vi "AlliGator Init Image Profile Window Menu.vi"(8 "error in":errorcluster, 11 "Menu in":refnum<k9>) -> (0 "error out":errorcluster)   [LabVIEW 2021, in "AlliGator Image Profile Window.lvlib"]
doc: "Initialize Profile Window menu."
uses:
  AlliGator Image Profile Window.lvlib
  AlliGator Variables List.ctl
  Image/Box Profile Type.ctl
  AlliGator Image Profile Intensity Type.ctl
  AlliGator Image Profile Average Intensity Type.ctl
  Variant/Variant to Data/Variant to Boolean.vi
  AlliGator Globals, Variables & Constants.lvlib
  Variant/Variant to Data/Variant to Data.lvlib
  Image/Image.lvlib
panel:
  # "see the AlliGator License on the block diagram (Ctrl+E or Window:Show Block Diagram)"
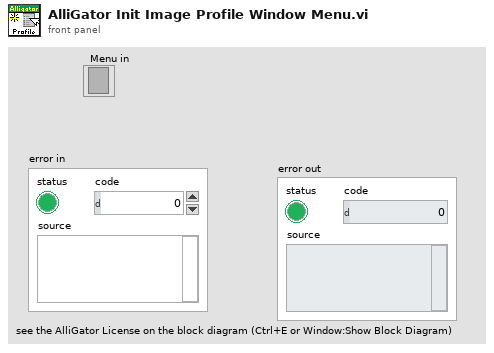
[diagram p1: front panel]
types:
  T1 = typedef "AlliGator Image Profile Window.lvlib/AlliGator Image Profile Average Intensity Type.ctl" = enum16{"Integrated Intensity", "Average Intensity", "Intensity-weighted Average Intensity"}
  T2 = typedef "AlliGator Image Profile Window.lvlib/AlliGator Image Profile Intensity Type.ctl" = enum16{"Raw Data", "Displayed Image", "Background-subtracted"}
  T3 = typedef "AlliGator Globals, Variables & Constants.lvlib/AlliGator Variables List.ctl" = enum16{"---- GUI ----", "Initialization Status", "State Indicators Refnum", "Original AlliGator Menu Items", "Current Action Loop State", "Script in progress", "Playback", "Loop Playback", "Search ROI Used", "Search ROI", "Decay Graph Max Legend Size", "Intensity Graph Max Legend Size", "Decay Statistics Graph Max Legend Size", "Phasor Graph Max Legend Size", "Phasor Ratio Graph Max Legend Size", "Lifetime Graph Max Legend Size", "---- Files ----", "Export Dataset Frames as Individual Files", "Show Batch Export Help Balloons", "Frames in Dataset", "ptu File Frame Start Indices", "Current Frame in Dataset", "Current Frame Timestamp", "------ Python Plugins ------", "Python Plugins Information", "Python Session", "Valid Python Session?", "---- Source Image ----", "Dataset Loaded", "Dataset Metadata", "Dataset Channel", "Dataset Data Description", "Background Dataset Metadata", "Background Dataset Channel", "Background Dataset Data Description", "Background File Subtraction", "Background File Path", "Background File Pile-up Correction", "Background File Pixel Well Capacity", "Background File Scaling Factor", "Source Image ROIs", "Current Source Image ROI", "Source Image ROI Event Refnum", "X_Source Image Display Range", "X_Source Image Palette Information", "Source Image Palette List", "Source Image Scale", "Current Dataset Load Settings", "Source Image:ROI Overlay Color", "---- Image Profile Window ----", "Image Profile:Overlay ROI in Source Image", "Image Profile Window Event Refnum", "Image Profile:IntensityType", "Image Profile:Intensity Average Type", "Image Profile:Intensity-weighted SDV", "Image Profile:Box Profile Type", "Image Profile Window Open", "Image Profile:Plotted Fit Parameter", "X_Type of Displayed Image", "X_Time Gate Slider", "Dataset Path", "Source Image Overlay to Erase", "Is Displayed Image Accumulated", "White Light Image Modified", "Mask Image Modified", "Macrotime Gate Separation", "------ Phasor Graph -------", "Phasor Graph:Show Line", "---- Phasor Plot ---", "Phasor Plot Parameters Changed", "FLI Dataset Modified since last Phasor Plot Calculation", "Phasor Harmonics Data", "Selected Phasor Harmonics", "Phasor Harmonic Manager Event Refnum", "Phasor Plot ROIs", "Current Phasor Plot ROI", "Phasor Plot ROI Event Refnum", "Phasor Plot Image Reference Points", "Phasor Plot Computed", "Phasor Plot Palette Information", "Phasor Plot Palette List", "Phasor Ratio Palette Information", "Phasor Ratio Palette List", "Phasor Image Scale", "Phasor Plot Image Overlay to Erase", "Phasor Plot Image Elements to Update", "Current Phasor Plot Calculation Parameters", "Current Phasor Calibration Options", "Reset Cumulated Phasor Plot", "Phasor Ratio Reference 1", "Phasor Ratio Lifetime Reference 1", "Phasor Ratio Reference 1 Frequency", "Phasor Ratio Reference 2", "Phasor Ratio Lifetime Reference 2", "Phasor Ratio Reference 2 Frequency", "---- Decay Analysis ----", "Number of Selected Decays to Fit", "LS Fit Results", "LAR Fit Results", "BS Fit Results", "Last Decay Max - Min", "Best Fit Parameters", "Best Fit Parameter Names", "Actual Size X", "Actual Size Y", "Binning X", "Binning Y", "Actual # Gates", "Dataset Number", "Gates to...", "Gates Skipped", "Gates to keep", "Gate Step", "Gate Separation", "Reversed Gates", "Pile-up Correction", "Pixel Well Capacity", "Background Subtracted", "Background Subtraction Method", "Background Definition Range", "Background File (deprecated)", "Number of Dataset Accumulated", "Array of Accumulated Dataset Paths", "Do Averaged Datasets", "Destination File Path", "Process Plot Target", "Use 1/D as Phasor Frequency", "---- Decay Fit Parameter Map -----", "Decay Fit Parameter Map Palette Information", "Decay Fit Parameter Map Palette List", "Local Decay Graph Window Event Refnum", "------- Local Decay Window ---------", "Use normalized IRF for convolution", "----- Miscellaneous ----", "Skippable Dialog Windows Status"}
  T4 = typedef "Image.lvlib/Box Profile Type.ctl" = enum16{"Full Width", "Half Width"}
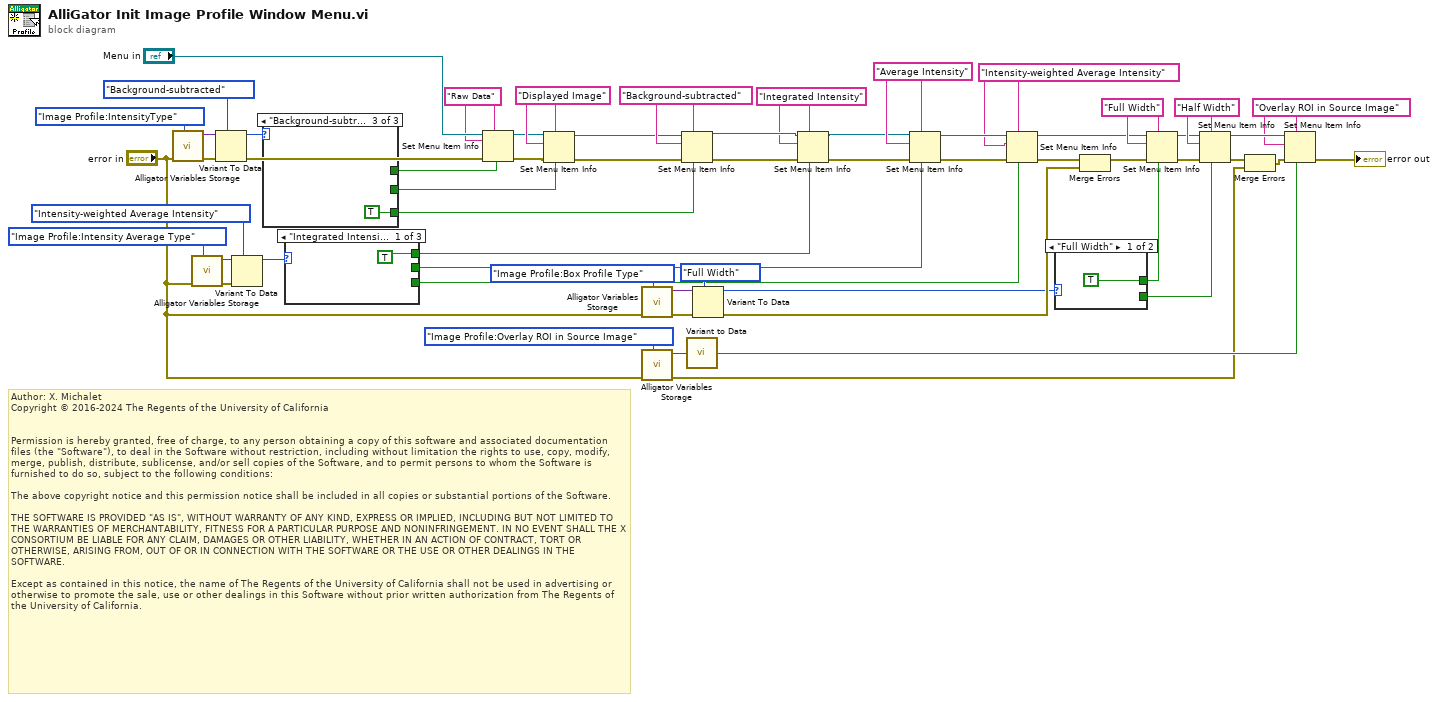
[diagram p0: block diagram]
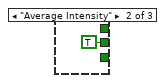
[diagram p2: hidden frame]
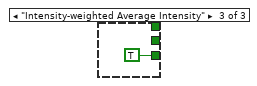
[diagram p3: hidden frame]
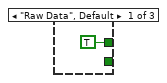
[diagram p4: hidden frame]
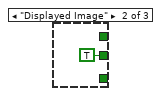
[diagram p5: hidden frame]
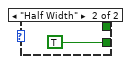
[diagram p6: hidden frame]
diagram:
  w2 = "Integrated Intensity" ("item tag")
  w13 = "Intensity-weighted Average Intensity" ("ItemTag")
  w14 = "Average Intensity" ("ItemTag")
  w34 = "Overlay ROI in Source Image" ("item tag")
  w55 = "Half Width" ("item tag")
  w54 = "Full Width" ("item tag")
  w50 = "Background-subtracted" ("ItemTag")
  w40 = "Raw Data" ("ItemTag")
  w41 = "Displayed Image" ("ItemTag")
  # "Author: X. Michalet\nCopyright © 2016-2024 The Regents of the University of California\n \n\nPermission is hereby granted, free of charge, to any person obtaining a copy of this software and associated documentation files (the \"Software\"), to deal in the Software without restriction, including without limitation the rights to use, copy, modify, merge, publish, distribute, sublicense, and/or sell copies of the Software, and to permit persons to whom the Software is furnished to do so, subject to the following conditions:\n\nThe above copyright notice and this permission notice shall be included in all copies or substantial portions of the Software.\n\nTHE SOFTWARE IS PROVIDED \"AS IS\", WITHOUT WARRANTY OF ANY KIND, EXPRESS OR IMPLIED, INCLUDING BUT NOT LIMITED TO THE WARRANTIES OF MERCHANTABILITY, FITNESS FOR A PARTICULAR PURPOSE AND NONINFRINGEMENT. IN NO EVENT SHALL THE X CONSORTIUM BE LIABLE FOR ANY CLAIM, DAMAGES OR OTHER LIABILITY, WHETHER IN AN ACTION OF CONTRACT, TORT OR OTHERWISE, ARISING FROM, OUT OF OR IN CONNECTION WITH THE SOFTWARE OR THE USE OR OTHER DEALINGS IN THE SOFTWARE.\n\nExcept as contained in this notice, the name of The Regents of the University of California shall not be used in advertising or otherwise to promote the sale, use or other dealings in this Software without prior written authorization from The Regents of the University of California."
  n1 = call "Alligator Variables Storage.vi"("AlliGator Variable"=AlliGator_Variables_List."Image Profile:IntensityType" ("Alligator Variable"), "Error In"="error in") -> ("Error Out"=w38:errorcluster, "Data out"=w24:variant)  [unwired: 7 in, 1 out]
  n2 = call "Alligator Variables Storage.vi"("AlliGator Variable"=AlliGator_Variables_List."Image Profile:Intensity Average Type" ("Alligator Variable"), "Error In"="error in") -> ("Error Out"=w11:errorcluster, "Data out"=w12:variant)  [unwired: 7 in, 1 out]
  n3 = Variant To Data(error in=w38, type=AlliGator_Image_Profile_Intensity_Type."Background-subtracted" ("Image Profile Intensity Type"), Variant=w24) -> (data=w22:T2, error out=w25:errorcluster)
  n4 = Variant To Data(error in=w11, type=AlliGator_Image_Profile_Average_Intensity_Type."Intensity-weighted Average Intensity" ("Image Profile Average Intenisty Type"), Variant=w12) -> (data=w10:T1)  [unwired: 1 out]
  n5 = case shown="\"Background-subtracted\"" w22 {
    tunnel: [TRUE ("checked") _ _] -> w21
    tunnel: [_ TRUE ("checked") _] -> w20
    tunnel: [_ _ TRUE ("checked")] -> w19
    frame "Raw Data", Default {
    }
    frame "Displayed Image" {
    }
    frame "Background-subtracted" {
    }
  }
  n6 = case shown="\"Integrated Intensity\", Default" w10 {
    tunnel: [_ TRUE ("checked") _] -> w8
    tunnel: [_ _ TRUE ("checked")] -> w7
    tunnel: [TRUE ("checked") _ _] -> w1
    frame "Integrated Intensity", Default {
    }
    frame "Average Intensity" {
    }
    frame "Intensity-weighted Average Intensity" {
    }
  }
  n7 = Set Menu Item Info(6:w21, 7:w40, 8:w25, 10:w40, 11:"Menu in") -> (0:w27:errorcluster, 3:w26:refnum<k9>)  [unwired: 2 in]
  n8 = Set Menu Item Info(6:w20, 7:w41, 8:w27, 10:w41, 11:w26) -> (0:w47:errorcluster, 3:w48:refnum<k9>)  [unwired: 2 in]
  n9 = call "Alligator Variables Storage.vi"("AlliGator Variable"=AlliGator_Variables_List."Image Profile:Box Profile Type" ("Alligator Variable"), "Error In"="error in") -> ("Error Out"=w44:errorcluster, "Data out"=w43:variant)  [unwired: 7 in, 1 out]
  n10 = call "Alligator Variables Storage.vi"("AlliGator Variable"=AlliGator_Variables_List."Image Profile:Overlay ROI in Source Image" ("Alligator Variable"), "Error In"="error in") -> ("Error Out"=w28:errorcluster, "Data out"=w32:variant)  [unwired: 7 in, 1 out]
  n11 = Set Menu Item Info(6:w19, 7:w50, 8:w47, 10:w50, 11:w48) -> (0:w4:errorcluster, 3:w6:refnum<k9>)  [unwired: 2 in]
  n12 = call-poly "Variant to Data.vi"("Variant"=w32) -> ("Value"=w30:bool)  [unwired: 8 in]
  n13 = Variant To Data(error in=w44, type=Box_Profile_Type."Full Width", Variant=w43) -> (data=w57:T4, error out=w59:errorcluster)
  n14 = Set Menu Item Info(6:w1, 7:w2, 8:w4, 10:w2, 11:w6) -> (0:w3:errorcluster, 3:w5:refnum<k9>)  [unwired: 2 in]
  n15 = Set Menu Item Info(6:w8, 7:w14, 8:w3, 10:w14, 11:w5) -> (0:w17:errorcluster, 3:w18:refnum<k9>)  [unwired: 2 in]
  n16 = Set Menu Item Info(6:w7, 7:w13, 8:w17, 10:w13, 11:w18) -> (0:w15:errorcluster, 3:w16:refnum<k9>)  [unwired: 2 in]
  n17 = case shown="\"Full Width\"" w57 {
    tunnel: [TRUE ("checked") _] -> w51
    tunnel: [_ TRUE ("checked")] -> w53
    frame "Full Width" {
    }
    frame "Half Width" {
    }
  }
  n18 = Merge Errors(w15, w59) -> (w58:errorcluster)
  n19 = Set Menu Item Info(6:w51, 7:w54, 8:w58, 10:w54, 11:w16) -> (0:w56:errorcluster, 3:w52:refnum<k9>)  [unwired: 2 in]
  n20 = Set Menu Item Info(6:w53, 7:w55, 8:w56, 10:w55, 11:w52) -> (0:w37:errorcluster, 3:w35:refnum<k9>)  [unwired: 2 in]
  n21 = Merge Errors(w37, w28) -> (w29:errorcluster)
  n22 = Set Menu Item Info(6:w30, 7:w34, 8:w29, 10:w34, 11:w35) -> (0:→"error out":errorcluster)  [unwired: 2 in, 1 out]
